vi "sum_alu.vi"(2 "INPUT_B":T1, 3 "INPUT_A":T1) -> (0 "OUTPUT":T2, 1 "OVERFLOW":bool)   [LabVIEW 2013]
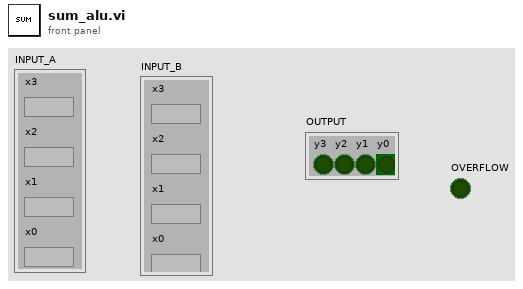
[diagram p1: front panel]
types:
  T1 = cluster{"x3":bool, "x2":bool, "x1":bool, "x0":bool}
  T2 = cluster{"y3":bool, "y2":bool, "y1":bool, "y0":bool}
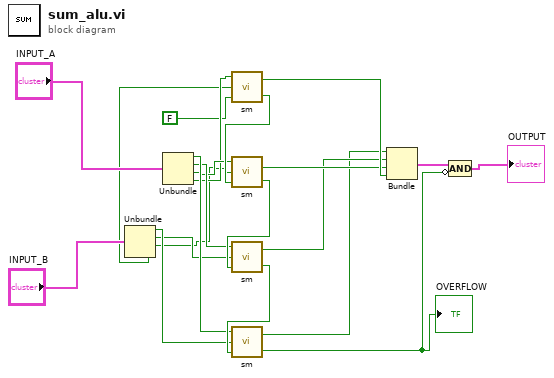
[diagram p0: block diagram]
diagram:
  n1 = Unbundle("INPUT_B") -> ("x3"=w12:bool, "x2"=w11:bool, "x1"=w10:bool, "x0"=w9:bool)
  n2 = Unbundle("INPUT_A") -> ("x3"=w16:bool, "x2"=w15:bool, "x1"=w14:bool, "x0"=w13:bool)
  n3 = call "sm.vi"("c"=FALSE, "b"=w9, "a"=w13) -> ("C"=w19:bool, "S"=w7:bool)
  n4 = call "sm.vi"("c"=w19, "b"=w10, "a"=w14) -> ("C"=w18:bool, "S"=w6:bool)
  n5 = call "sm.vi"("c"=w18, "b"=w11, "a"=w15) -> ("C"=w17:bool, "S"=w5:bool)
  n6 = call "sm.vi"("c"=w17, "b"=w12, "a"=w16) -> ("C"=w2:bool, "S"=w4:bool)
  "OVERFLOW" <- w2
  n7 = Bundle("S"=w4, "S"=w5, "S"=w6, "S"=w7) -> (w3:cluster{"S":bool, "S":bool, "S":bool, "S":bool})  [unwired: 1 in]
  n8 = Compound Arithmetic op=AND(w3, invert w2) -> (→"OUTPUT":cluster{"S":bool, "S":bool, "S":bool, "S":bool})
